vi "Not.vi"(3 "in":bool) -> (1 "out":bool)   [LabVIEW 2014]
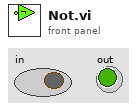
[diagram p1: front panel]
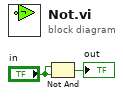
[diagram p0: block diagram]
diagram:
  n1 = Not And(1:"in", 2:"in") -> (0:→"out":bool)
